vi "Ping.vi"(8 "error in (no error)":errorcluster, 11 "MicronManager in":refnum<class "MicronManager.lvclass">) -> (0 "error out":errorcluster, 2 "Responses":string[](array[string]), 3 "MicronManager out":refnum<class "MicronManager.lvclass">)   [LabVIEW 2019, in "MicronManager.lvclass"]
uses:
  MicronManager.lvclass
  MicronManager.lvclass/MicronManager.ctl
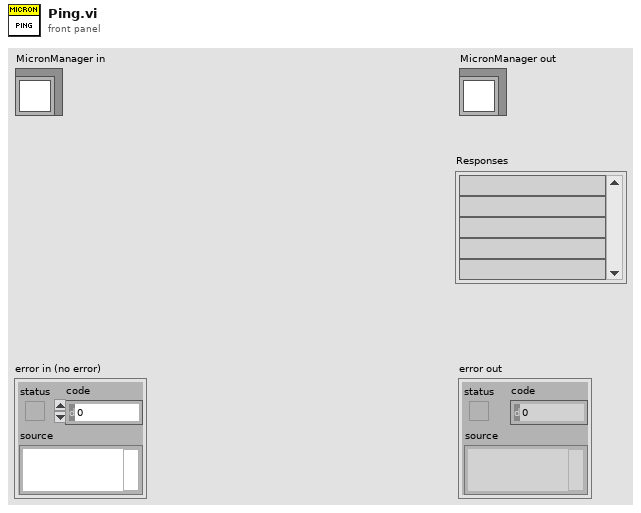
[diagram p1: front panel]
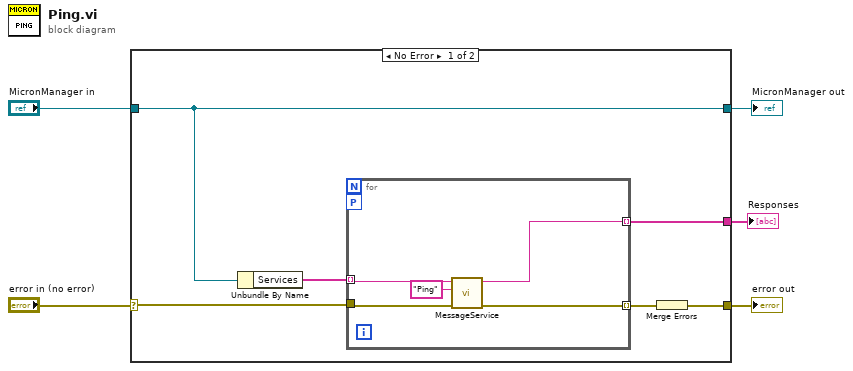
[diagram p0: block diagram]
diagram:
  n1 = case shown="No Error" "error in (no error)" {
    selector: "error in (no error)" -> [w9 w18]
    tunnel: [w7 w18] -> w4
    tunnel: [w10 w17] -> w2
    tunnel: "MicronManager in" -> [w10 w17]
    tunnel: [w6 _] -> w1
    frame No Error {
      n2 = Unbundle By Name(w10) -> ("Services"=w11:string[])
      n3 = for {
        tunnel: w11 -> [w14] mode=indexing
        tunnel: [w15] -> w8 mode=indexing
        tunnel: [w12] -> w6 mode=indexing
        tunnel: w9 -> [w16]
        workers-P: _ -> [_]
        n4 = call "MessageService.vi"("error in (no error)"=w16, "Message"="Ping", "Service Name"=w14) -> ("error out"=w15:errorcluster, "Response"=w12:string)  [unwired: 7 in]
      }
      n5 = Merge Errors(w8) -> (w7:errorcluster)
    }
    frame Error {
    }
  }
  "error out" <- w4
  "MicronManager out" <- w2
  "Responses" <- w1
